vi "Static.vi"() -> ()   [LabVIEW 2023, in "Panel Actor.lvlib" / "Panel.lvlib" / "Panel Registry.lvclass"]
uses:
  Panel Registry.lvclass
panel:
  out "Last Event":variant
  out "Panel State":variant
  out "Event Lookup":variant
  out "Parent Lookup":variant
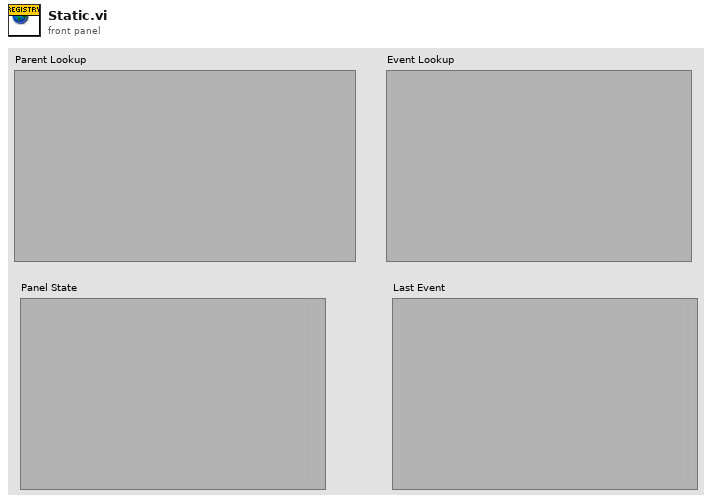
[diagram p1: front panel]
diagram:
